vi "New Application.vi"(8 "error in (no error)":errorcluster) -> (0 "error out":errorcluster, 3 "Application":refnum<data-value>)   [LabVIEW 2015, in "Application.lvclass"]
uses:
  Application.lvclass
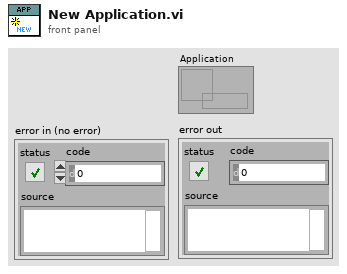
[diagram p1: front panel]
types:
  T1 = typedef "Application Config Typedef.ctl" = cluster{"Auto Load Project":bool, "Project Path":string, "Plugin Folders":string}
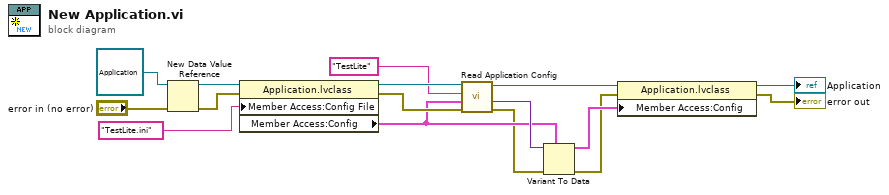
[diagram p0: block diagram]
diagram:
  n1 = New Data Value Reference(data value=refnum<class "Application.lvclass"> refnum ("Application.lvclass"), error in="error in (no error)") -> (data value reference=w14:refnum<data-value>, error out=w13:errorcluster)
  n2 = property class="Application.lvclass"(reference=w14, error in=w13, "Member Access:Config File"="TestLite.ini" ("Config File")) -> (reference out=w11:refnum<data-value>, error out=w10:errorcluster, "Member Access:Config"=w6:T1)
  n3 = call "Read Application Config.vi"("error in (no error)"=w10, "Config Type In"=w6, "Section"="TestLite", "Application in"=w11) -> ("error out"=w5:errorcluster, "Config Data out"=w7:variant, "Application out"=w8:refnum<data-value>)  [unwired: 5 in]
  n4 = Variant To Data(error in=w5, type=w6, Variant=w7) -> (data=w4:T1, error out=w3:errorcluster)
  n5 = property class="Application.lvclass"(reference=w8, error in=w3, "Member Access:Config"=w4) -> (reference out=→"Application":refnum<data-value>, error out=→"error out":errorcluster)
